vi "Handle_counter_bottle_drop.vi"(10 "Available Data Names":string[](array[string]), 11 "ListBox in":refnum<vi>) -> (3 "Boolean":bool)   [LabVIEW 2016]
uses:
  <vilib>/regexp/Match Regular Expression.xnode
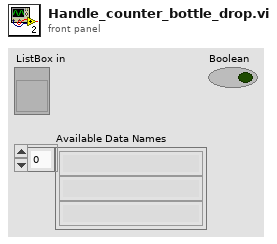
[diagram p1: front panel]
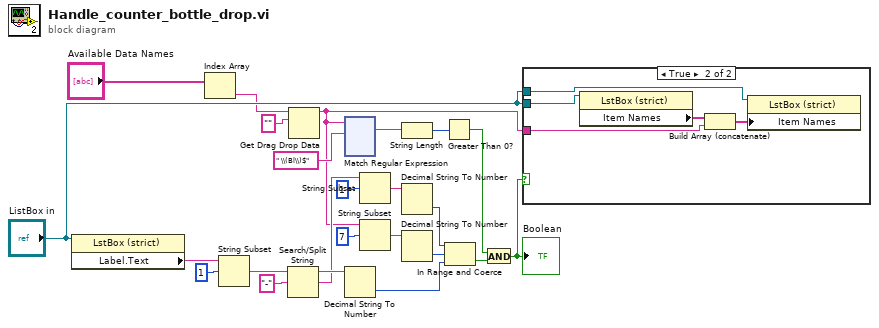
[diagram p0: block diagram]
diagram:
  n1 = property class="LstBox (strict)"(reference="ListBox in") -> ("Label.Text"=w7:string)  [unwired: 1 in, 2 out]
  n2 = Index Array(array="Available Data Names") -> (element=w17:string)  [unwired: 1 in]
  n3 = String Subset(string=w7, offset (0)=1) -> (substring=w10:string)  [unwired: 1 in]
  n4 = Search/Split String(string=w10, search string/char (-)="-") -> (substring before match=w13:string, match + rest of string=w12:string)  [unwired: 1 in, 1 out]
  n5 = Get Drag Drop Data(8:"" ("type"), 9:w17) -> (3:w2:string)  [unwired: 1 in, 1 out]
  n6 = xnode "Match Regular Expression"("input string"=w2, "regular expression"=" \\(Bl\\)$") -> ("whole match"=w4:string)  [unwired: 4 in, 4 out]
  n7 = Decimal String To Number(string=w13) -> (number=w16:i32)  [unwired: 2 in, 1 out]
  n8 = String Subset(string=w12, offset (0)=1) -> (substring=w14:string)  [unwired: 1 in]
  n9 = String Subset(string=w2, offset (0)=7) -> (substring=w20:string)  [unwired: 1 in]
  n10 = String Length(string=w4) -> (length=w3:i32)
  n11 = Decimal String To Number(string=w14) -> (number=w15:i32)  [unwired: 2 in, 1 out]
  n12 = Decimal String To Number(string=w20) -> (number=w21:i32)  [unwired: 2 in, 1 out]
  n13 = Greater Than 0?(x=w3) -> (x > 0?=w1:bool)
  n14 = In Range and Coerce(upper limit=w15, x=w21, lower limit=w16) -> (In Range?=w22:bool)  [unwired: 1 out]
  n15 = And(x=w1, y=w22) -> (x .and. y?=w23:bool)
  "Boolean" <- w23
  n16 = case shown="True" w23 {
    tunnel: w2 -> [_ w27]
    tunnel: "ListBox in" -> [_ w26]
    tunnel: "ListBox in" -> [_ w25]
    frame False {
    }
    frame True {
      n17 = property class="LstBox (strict)"(reference=w26) -> ("Item Names"=w29:string[])  [unwired: 1 in, 2 out]
      n18 = Build Array (concatenate)(w29, w27) -> (w28:string[])
      n19 = property class="LstBox (strict)"(reference=w25, "Item Names"=w28) -> ()  [unwired: 1 in, 2 out]
    }
  }
